vi "Equalize.vi"(11 "Analog Waveform Array in":waveform(dbl)[](array[waveform])) -> (1 "Target dt":dbl, 3 "Analog Waveform Array out":waveform(dbl)[](array[waveform]))   [LabVIEW 2018, in "Waveform Equalizer.lvlib"]
uses:
  Waveform Equalizer.lvlib
  subVIs/Interpolate.vi
  subVIs/Greater or Equal with Epsilon.vi
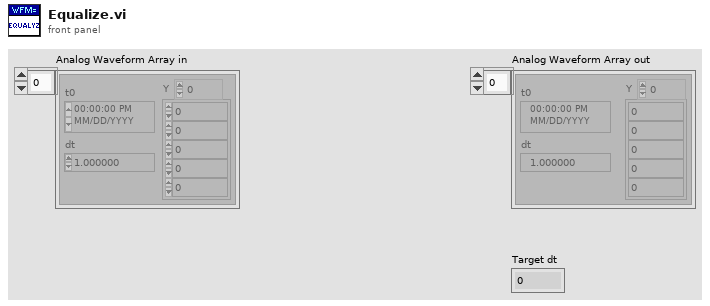
[diagram p1: front panel]
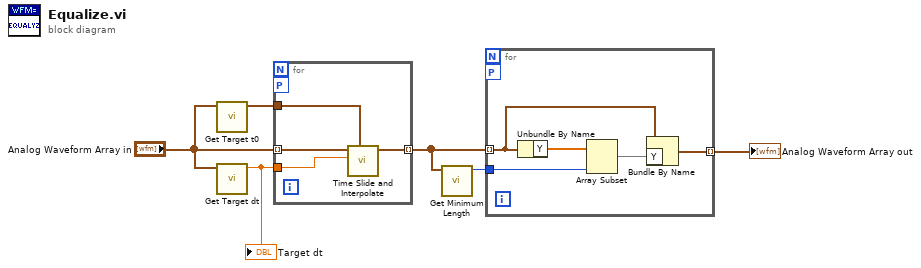
[diagram p0: block diagram]
diagram:
  n1 = call "Get Target t0.vi"("Analog Waveform Array in"="Analog Waveform Array in") -> ("Target t0"=w4:timestamp)  [unwired: 10 in]
  n2 = call "Get Target dt.vi"("Analog Waveform Array in"="Analog Waveform Array in") -> ("Target dt"=w3:dbl)  [unwired: 10 in]
  "Target dt" <- w3
  n3 = for {
    tunnel: "Analog Waveform Array in" -> [w10] mode=indexing
    tunnel: w4 -> [w9]
    tunnel: w3 -> [w8]
    tunnel: [w7] -> w2 mode=indexing
    workers-P: _ -> [_]
    n4 = call "Time Slide and Interpolate.vi"("Target t0"=w9, "Target dt"=w8, "input waveform"=w10) -> ("output waveform"=w7:waveform(dbl))  [unwired: 8 in]
  }
  n5 = call "Get Minimum Length.vi"("Analog Waveform Array in"=w2) -> ("Target Length"=w1:i32)  [unwired: 10 in]
  n6 = for {
    tunnel: w2 -> [w13] mode=indexing
    tunnel: w1 -> [w12]
    tunnel: [w11] -> w6 mode=indexing
    workers-P: _ -> [_]
    n7 = Unbundle By Name(w13) -> ("Y"=w15:dbl[])
    n8 = Array Subset(array=w15, length=w12) -> (w14:dbl[])  [unwired: 1 in]
    n9 = Bundle By Name(cluster=w13, "Y"=w14) -> (w11:waveform(dbl))
  }
  "Analog Waveform Array out" <- w6
